vi "Instr_InitObject.vi"(8 "error in (no error)":errorcluster, 9 "Instrument Configuration":variant, 10 "GPIB Address":string, 11 "HP4284 in":refnum<class "HP4284.lvclass">) -> (0 "error out":errorcluster, 3 "HP4284 out":refnum<class "HP4284.lvclass">)   [LabVIEW 2018, in "HP4284.lvclass"]
uses:
  HP4284.lvclass
  InstrumentSetup.vi
  HP4284A_CommandsGlobal.vi
  LCRControl.lvclass
  InstrControl.lvclass
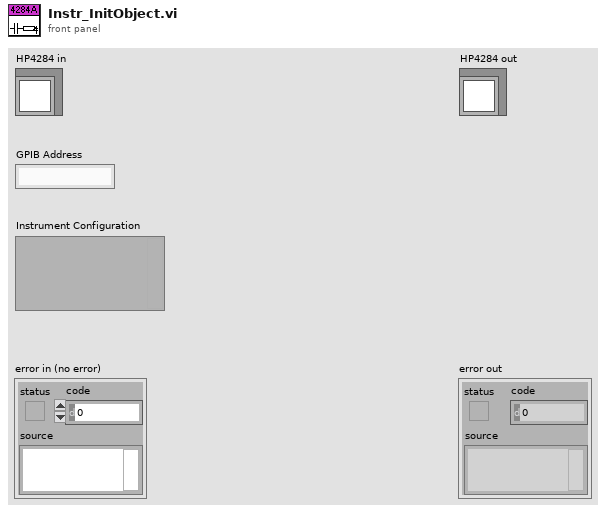
[diagram p1: front panel]
types:
  T1 = cluster{"RC Configuration":u16, "AC amplitude [V]":dbl, "AC frequency [Hz]":i32, "HP4284.lvclass":refnum<class "HP4284.lvclass">}
  T2 = cluster{"Instrument name":string, "Instrument type":u16, "Command \"Initialise LCR\"":string, "Command \"OC Trim\"":string, "Command \"LCR Readout\"":string}
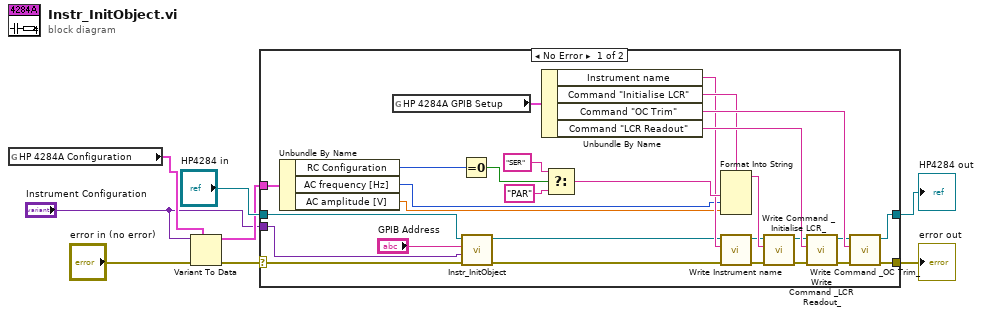
[diagram p0: block diagram]
diagram:
  n1 = global read "InstrumentSetup.vi" "HP 4284A Configuration"() -> (w7:T1)
  n2 = Variant To Data(error in="error in (no error)", type=w7, Variant="Instrument Configuration") -> (data=w3:T1, error out=w2:errorcluster)
  n3 = case shown="No Error" w2 {
    selector: w2 -> [w21 w38]
    tunnel: [w31 w38] -> w5
    tunnel: [w32 w37] -> w4
    tunnel: "HP4284 in" -> [w22 w37]
    tunnel: w3 -> [w14 _]
    tunnel: "Instrument Configuration" -> [w9 _]
    frame No Error {
      n4 = Unbundle By Name(w14) -> ("RC Configuration"=w13:u16, "AC frequency [Hz]"=w11:i32, "AC amplitude [V]"=w12:dbl)
      n5 = global read "HP4284A_CommandsGlobal.vi" "HP 4284A GPIB Setup"() -> (w10:T2)
      n6 = Equal To 0?(x=w13) -> (x = 0?=w28:bool)
      n7 = call-parent "Instr_InitObject.vi"("error in (no error)"=w21, "Instrument Configuration"=w9, "GPIB Address"="GPIB Address", "LCRControl in"=w22) -> ("error out"=w19:errorcluster, "LCRControl out"=w17:refnum<class "HP4284.lvclass">)  [unwired: 6 in]
      n8 = Unbundle By Name(w10) -> ("Instrument name"=w20:string, "Command \"Initialise LCR\""=w24:string, "Command \"OC Trim\""=w35:string, "Command \"LCR Readout\""=w36:string)
      n9 = Select(t="SER", s=w28, f="PAR") -> (s? t:f=w25:string)
      n10 = Format Into String(format string=w24, w25, w11, w12) -> (resulting string=w23:string)  [unwired: 2 in, 1 out]
      n11 = call-dynamic "Write Instrument name.vi"("error in (no error)"=w19, "Instrument name"=w20, "InstControl in"=w17) -> ("error out"=w18:errorcluster, "InstControl out"=w16:refnum<class "HP4284.lvclass">)  [unwired: 7 in]
      n12 = call-dynamic "Write Command _Initialise LCR_.vi"("error in (no error)"=w18, "Command \"Initialise LCR\""=w23, "LCRControl in"=w16) -> ("error out"=w30:errorcluster, "LCRControl out"=w34:refnum<class "HP4284.lvclass">)  [unwired: 7 in]
      n13 = call-dynamic "Write Command _LCR Readout_.vi"("error in (no error)"=w30, "Command \"LCR Readout\""=w36, "LCRControl in"=w34) -> ("error out"=w29:errorcluster, "LCRControl out"=w33:refnum<class "HP4284.lvclass">)  [unwired: 7 in]
      n14 = call-dynamic "Write Command _OC Trim_.vi"("error in (no error)"=w29, "Command \"OC Trim\""=w35, "LCRControl in"=w33) -> ("error out"=w31:errorcluster, "LCRControl out"=w32:refnum<class "HP4284.lvclass">)  [unwired: 7 in]
    }
    frame Error {
    }
  }
  "error out" <- w5
  "HP4284 out" <- w4
